vi "Get Log Text.vi"(8 "error in (no error)":errorcluster, 11 "Event_TextLog in":refnum<class "Event_TextLog.lvclass">) -> (0 "error out":errorcluster, 2 "Log Message":string, 3 "Event_TextLog out":refnum<class "Event_TextLog.lvclass">)   [LabVIEW 2021, in "Event_TextLog.lvclass"]
uses:
  Event_TextLog.lvclass
  Event_TextLog.lvclass/Event_TextLog.ctl
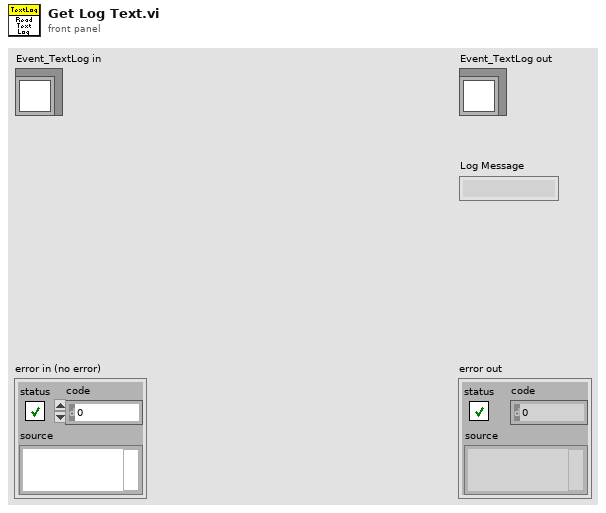
[diagram p1: front panel]
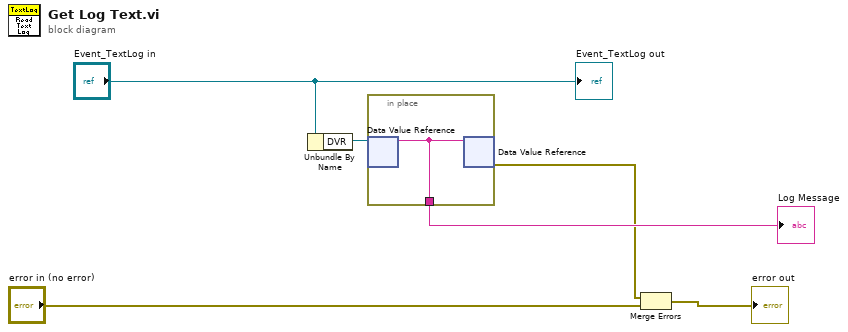
[diagram p0: block diagram]
diagram:
  n1 = Unbundle By Name("Event_TextLog in") -> ("DVR"=w1:refnum<data-value>)
  n2 = in-place {
    in-place-border: [w7] -> w3
    n3 = in-place-dvr #1(w1) -> (w7:string)  [unwired: 1 out]
    n4 = in-place-dvr #1(w7) -> (w2:errorcluster)  [unwired: 1 out]
  }
  "Log Message" <- w3
  n5 = Merge Errors(w2, "error in (no error)") -> (→"error out":errorcluster)
  "Event_TextLog out" <- "Event_TextLog in"
